vi "Elevator Controller.vi"(8 "error in":errorcluster) -> ()   [LabVIEW 2017]
doc: "This VI executes continuously carrying out the current operation and responding to updates or new operations. It will often contain the timing or control code that is difficult to place directly in TeleOp. This VI generally opens all sensors and motors and isolates the rest of the robot code from knowing how the operations are carried out."
uses:
  <vilib>/Rock Robotics/WPI/Framework/Completion Status.ctl
  Elevator Setpoints.ctl
  Elevator Operations.ctl
  <vilib>/Rock Robotics/WPI/ThirdParty/Phoenix-LabVIEW/Motor Controller/Controls/CTRE_Phoenix_MotorControl_FeedbackDevice.ctl
  <vilib>/Rock Robotics/WPI/ThirdParty/Phoenix-LabVIEW/Motor Controller/Controls/CTRE_Phoenix_MotorControl_LimitSwitchSource_Local.ctl
  <vilib>/Rock Robotics/WPI/ThirdParty/Phoenix-LabVIEW/Motor Controller/Controls/CTRE_Phoenix_MotorControl_LimitSwitchNormal.ctl
  <vilib>/Rock Robotics/WPI/ThirdParty/Phoenix-LabVIEW/Motor Controller/Controls/CTRE_Phoenix_MotorControl_ControlMode.ctl
  <vilib>/Rock Robotics/WPI/ThirdParty/Phoenix-LabVIEW/Motor Controller/Get/CTRE_Phoenix_MotorController_GetOutputCurrent_Enhanced.vi
  <vilib>/Rock Robotics/WPI/ThirdParty/Phoenix-LabVIEW/Motor Controller/Get/CTRE_Phoenix_MotorController_GetVoltage.vi
  Support Code/Global Constants.vi
  <vilib>/Rock Robotics/WPI/ThirdParty/Phoenix-LabVIEW/Motor Controller/Get/CTRE_Phoenix_MotorController_GetSelectedSensorData.vi
  <vilib>/Rock Robotics/Network Tables/NT Write Boolean.vi
panel:
  out "Current":dbl=0.5
  out "Output":dbl=0.06256109481915934
  out "Current":dbl(graph)=0.5
  out "Output":dbl(graph)=0.06256109481915934
  in  "F":dbl=0.0095 format="%#_13g"
  in  "P":dbl=0.7 format="%#_13g"
  in  "Max Acceleration":i32=6000
  in  "Cruise Velocity":i32=6000
  in  "Interactive Values":T1={"Operation"=enum."Zero Elevator Encoders", "Setpoint"=2.0, "Duration"=0.0}
  out "Current\nCmd":string="Started at  09:56:44.845\n: Reserve,  S 0.0, D 0.000000"
  in  "Buttons":cluster{"Execute Cmd":bool, "Abort Cmd":bool}
  out "Command Timing":cluster{"Start Time (ms)":u32, "Iterations":i32}={"Start Time (ms)"=1100696, "Iterations"=0}
  out "Status":T3
  # "Interactive Command: You may fill in the settings for a command\nand schedule it with the Execute button. You can observe and abort\nany command while fine tuning the code for the controller."
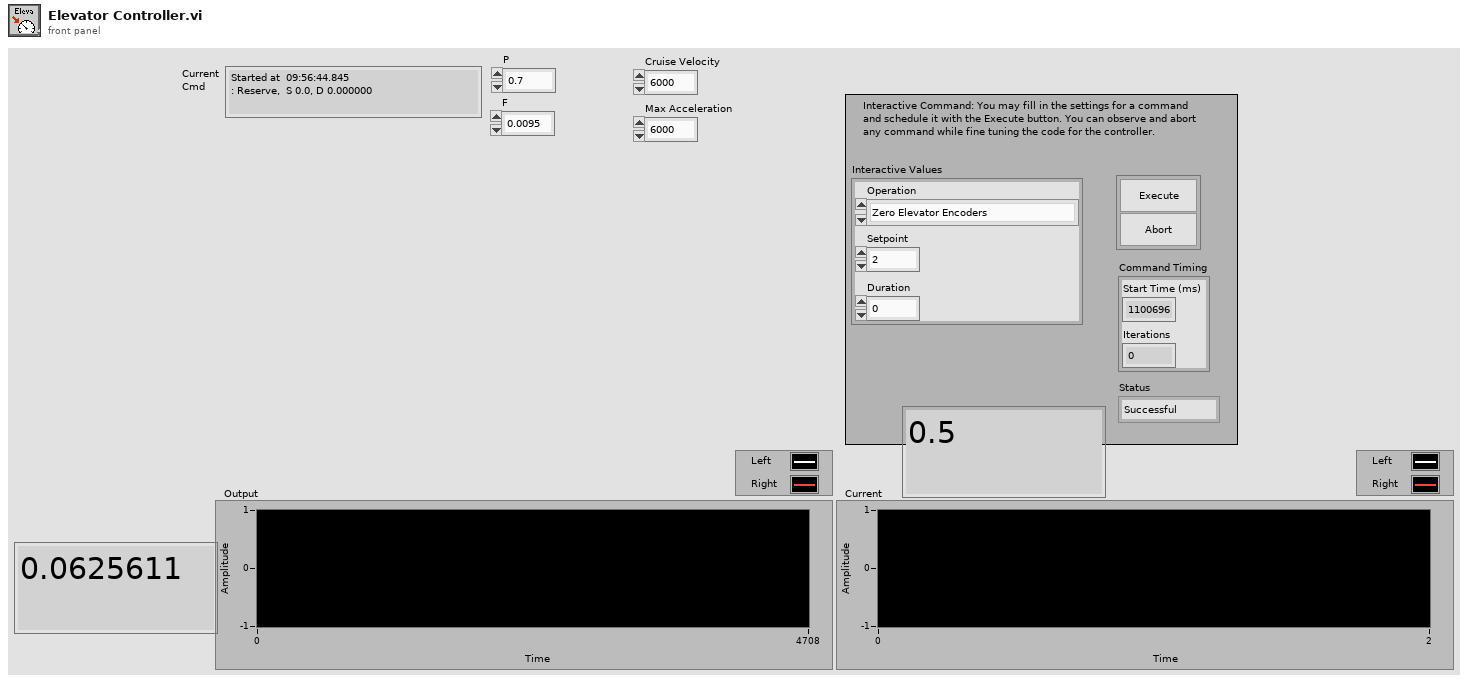
[diagram p1: front panel]
types:
  T1 = typedef "Elevator Setpoints.ctl" = cluster{"Operation":T2, "Setpoint":dbl, "Duration":dbl}
  T2 = typedef "Elevator Operations.ctl" = enum16{"Reserve", "Read Current", "Immediate", "Go to Height", "Fudge Up", "Fudge Down", "Zero Elevator Encoders", "Go to A", "Hold A", "Hold A for Duration"}
  T3 = typedef "Completion Status.ctl" = enum16{"Successful", "Aborted", "Incomplete"}
  T4 = typedef "CTRE_Phoenix_MotorControl_LimitSwitchNormal.ctl" = enum16{"Normally Open", "Normally Closed", "Disabled"}
  T5 = typedef "CTRE_Phoenix_MotorControl_LimitSwitchSource_Local.ctl" = enum16{"Feedback Connector", "Remote Talon SRX", "Remote CANifier", "Deactivated"}
  T6 = typedef "CTRE_Phoenix_MotorControl_FeedbackDevice.ctl" = i8
  T7 = typedef "WPI_MotorControlDeviceRef.ctl" = cluster{"DeviceStatus":errorcluster, "Type":T8, "PWM":cluster{"PWM Channel":T9, "DeadBand":T10}, "CAN":cluster{"Device Number":u8, "SetOutput VI Ref":variant, "GetOutput VI Ref":variant, "Enable VI Ref":variant, "Disable VI Ref":variant, "Data":variant}, "Invert":bool, "DIO PWM":cluster{"PWM \"Enable\" Channel":T9, "DIOChannel":T11, "PWM Rate":dbl}}
  T8 = typedef "WPI_MotorControlType.ctl" = enum16{"PWM", "CAN", "DIO PWM"}
  T9 = typedef "FPGA_DIOPWMChannel.ctl" = enum8{"PWM 0", "PWM 1", "PWM 2", "PWM 3", "PWM 4", "PWM 5", "PWM 6", "PWM 7", "PWM 8", "PWM 9", "PWM MXP 0", "PWM MXP 1", "PWM MXP 2", "PWM MXP 3", "PWM MXP 4", "PWM MXP 5", "PWM MXP 6", "PWM MXP 7", "PWM MXP 8", "PWM MXP 9", "Invalid"}
  T10 = typedef "WPI_PWMDeadband.ctl" = cluster{"Name":string, "maxPositivePwm":i32, "minPositivePwm":i32, "centerPwm":i32, "maxNegativePwm":i32, "minNegativePwm":i32, "angularRange":u16}
  T11 = typedef "FPGA_DIOChannel.ctl" = enum8{"DIO 0", "DIO 1", "DIO 2", "DIO 3", "DIO 4", "DIO 5", "DIO 6", "DIO 7", "DIO 8", "DIO 9", "DIO MXP 0", "DIO MXP 1", "DIO MXP 2", "DIO MXP 3", "DIO MXP 4", "DIO MXP 5", "DIO MXP 6", "DIO MXP 7", "DIO MXP 8", "DIO MXP 9", "DIO MXP 10", "DIO MXP 11", "DIO MXP 12", "DIO MXP 13", "DIO MXP 14", "DIO MXP 15", "SPI Port CS1", "SPI Port CS2", "SPI Port CS3", "SPI Port MISO", "SPI Port MOSI", "Invalid"}
  T12 = typedef "Command Status Info.ctl" = cluster{"Name":string, "Status":T3, "notifier out":T13}
  T13 = typedef "Completion Notifier.ctl" = refnum<notifier>
  T14 = cluster{"Current Command":T1, "Command Timing":cluster{"Start Time (ms)":u32, "Iterations":i32}, "Command Arguments":cluster{"Command Info":T12, "Description":string, "Default Command":T1, "queue out":refnum<queue>, "Subsystem Name":string}}
  T15 = typedef "CTRE_Phoenix_MotorControl_ControlMode.ctl" = u16
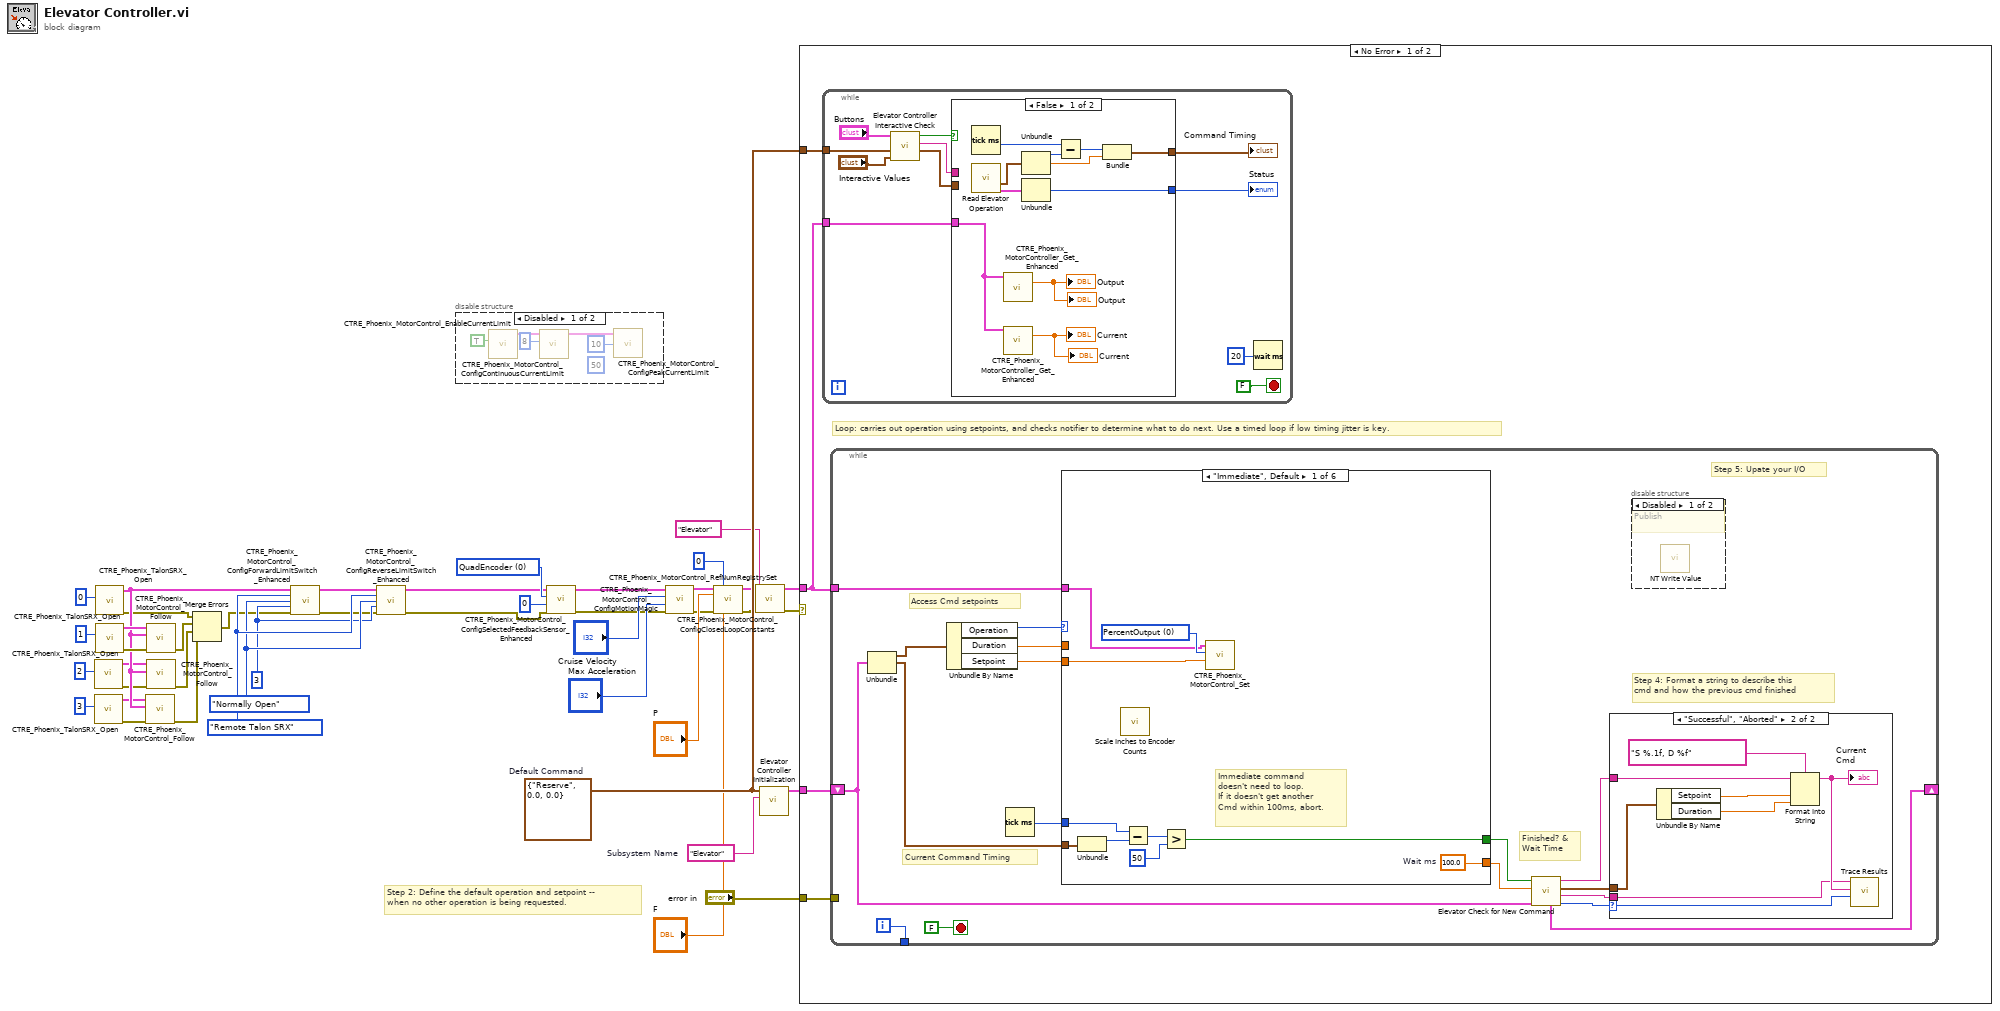
[diagram p0: block diagram]
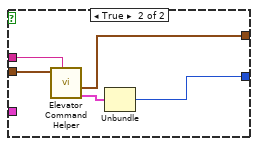
[diagram p2: hidden frame]
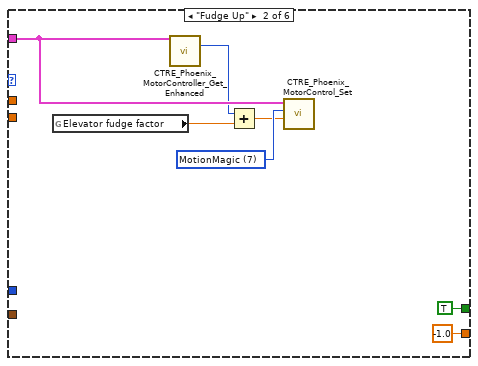
[diagram p5: hidden frame]
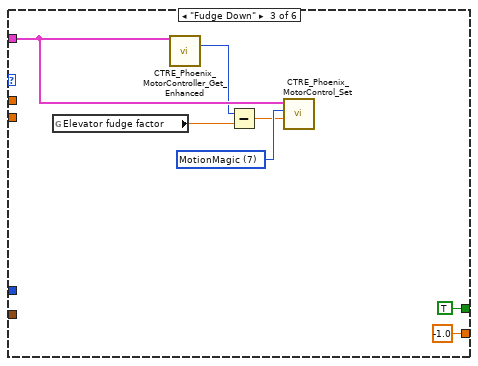
[diagram p6: hidden frame]
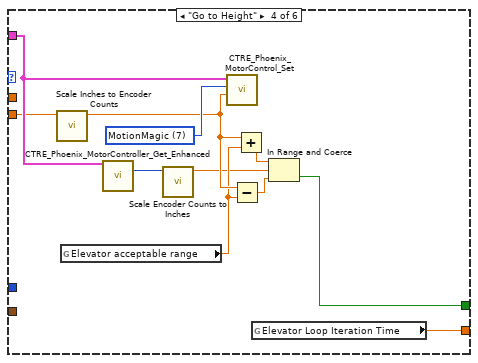
[diagram p7: hidden frame]
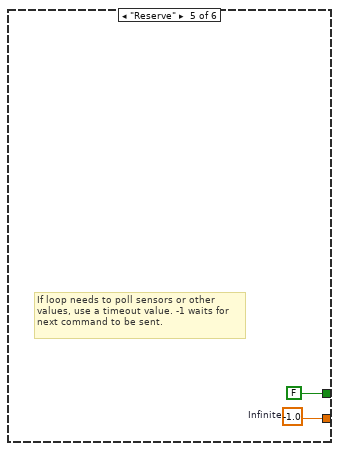
[diagram p8: hidden frame]
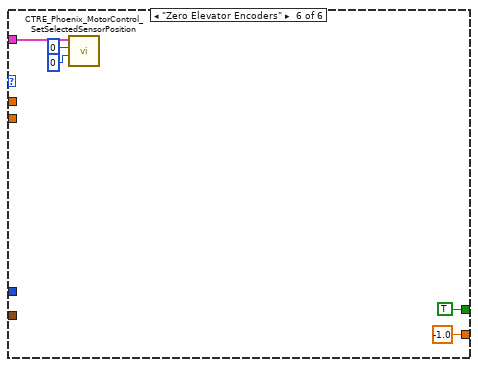
[diagram p9: hidden frame]
diagram:
  w21 = 3 ("deviceID")
  w22 = CTRE_Phoenix_MotorControl_LimitSwitchNormal."Normally Open" ("NormallyOpenOrClosed")
  w23 = CTRE_Phoenix_MotorControl_LimitSwitchSource_Local."Remote Talon SRX" ("Limit Switch Source")
  w27 = T6 0 items=["None"=-1, "QuadEncoder"=0, "Analog"=2, "Tachometer"=4, "Pulse Width Encoded Position"=8, "Sensor Sum (S0 + S1)"=9, "Sensor Difference (D0 - D1)"=10, "Remote Source 0"=11, "Remote Source 1"=12, "Software Emulated"=15] ("Feedback Device")
  w40 = T1 {"Operation"=enum."Reserve", "Setpoint"=0.0, "Duration"=0.0}  # Default Command
  w41 = "Elevator"  # Subsystem Name
  # "Step 2: Define the default operation and setpoint --\nwhen no other operation is being requested."
  n1 = call <vilib>:"CTRE_Phoenix_TalonSRX_Open.vi"("Device Number"=u8 2) -> ("error out"=w4:errorcluster, "CAN Talon SRX Ref"=w3:T7)  [unwired: 9 in]
  n2 = call <vilib>:"CTRE_Phoenix_TalonSRX_Open.vi"("Device Number"=u8 3) -> ("error out"=w2:errorcluster, "CAN Talon SRX Ref"=w1:T7)  [unwired: 9 in]
  n3 = call <vilib>:"CTRE_Phoenix_TalonSRX_Open.vi"("Device Number"=u8 0) -> ("error out"=w20:errorcluster, "CAN Talon SRX Ref"=w26:T7)  [unwired: 9 in]
  n4 = call <vilib>:"CTRE_Phoenix_TalonSRX_Open.vi"("Device Number"=u8 1) -> ("error out"=w30:errorcluster, "CAN Talon SRX Ref"=w29:T7)  [unwired: 9 in]
  n5 = call <vilib>:"CTRE_Phoenix_MotorControl_Follow.vi"("error in (no error)"=w2, "Master Controller to Follow"=w26, "PhoenixMotorControlDevRef"=w1) -> ("error out"=w17:errorcluster)  [unwired: 7 in, 1 out]
  n6 = call <vilib>:"CTRE_Phoenix_MotorControl_Follow.vi"("error in (no error)"=w30, "Master Controller to Follow"=w26, "PhoenixMotorControlDevRef"=w29) -> ("error out"=w19:errorcluster)  [unwired: 7 in, 1 out]
  n7 = call <vilib>:"CTRE_Phoenix_MotorControl_Follow.vi"("error in (no error)"=w4, "Master Controller to Follow"=w26, "PhoenixMotorControlDevRef"=w3) -> ("error out"=w18:errorcluster)  [unwired: 7 in, 1 out]
  n8 = Merge Errors(w20, w19, w18, w17) -> (w16:errorcluster)
  n9 = call <vilib>:"CTRE_Phoenix_MotorControl_ConfigForwardLimitSwitch_Enhanced.vi"("PhoenixMotorControlDevRef"=w26, "Limit Switch Source"=w23, "NormallyOpenOrClosed"=w22, "deviceID"=w21, "error in (no error)"=w16) -> ("PhoenixMotorControlDevRef"=w25:T7, "error out"=w15:errorcluster)  [unwired: 9 in]
  n10 = call <vilib>:"CTRE_Phoenix_MotorControl_ConfigReverseLimitSwitch_Enhanced.vi"("PhoenixMotorControlDevRef"=w25, "Limit Switch Source"=w23, "NormallyOpenOrClosed"=w22, "deviceID"=w21, "error in (no error)"=w15) -> ("PhoenixMotorControlDevRef"=w24:T7, "error out"=w14:errorcluster)  [unwired: 9 in]
  n11 = disable-structure shown="Disabled" {
    frame Disabled {
      (unwired) 50 ("Peak Current Maximum Duration (ms)")
      n12 = call <vilib>:"CTRE_Phoenix_MotorControl_EnableCurrentLimit.vi"("Enable Current Limit?"=TRUE) -> ("PhoenixMotorControlDevRef"=w47:T7)  [unwired: 9 in, 1 out]
      n13 = call <vilib>:"CTRE_Phoenix_MotorControl_ConfigContinuousCurrentLimit.vi"("Continuous Current Limit (Amps)"=8, "PhoenixMotorControlDevRef"=w47) -> ("PhoenixMotorControlDevRef"=w48:T7)  [unwired: 8 in, 1 out]
      n14 = call <vilib>:"CTRE_Phoenix_MotorControl_ConfigPeakCurrentLimit.vi"("Peak Current (Amps)"=10, "PhoenixMotorControlDevRef"=w48) -> ()  [unwired: 8 in, 2 out]
    }
    frame Enabled {
    }
  }
  n15 = call <vilib>:"CTRE_Phoenix_MotorControl_ConfigSelectedFeedbackSensor_Enhanced.vi"("error in (no error)"=w14, "pidLoopIdx"=0, "Feedback Device"=w27, "PhoenixMotorControlDevRef"=w24) -> ("error out"=w13:errorcluster, "PhoenixMotorControlDevRef"=w32:T7)  [unwired: 6 in]
  n16 = call <vilib>:"CTRE_Phoenix_MotorControl_ConfigMotionMagic.vi"("error in (no error)"=w13, "Acceleration"="Max Acceleration", "Cruise Velocity"="Cruise Velocity", "PhoenixMotorControlDevRef"=w32) -> ("error out"=w12:errorcluster, "PhoenixMotorControlDevRef"=w36:T7)  [unwired: 6 in]
  n17 = call <vilib>:"CTRE_Phoenix_MotorControl_ConfigClosedLoopConstants.vi"("PhoenixMotorControlDevRef"=w36, "slotIdx"=0, "P"="P", "error in (no error)"=w12, "F"="F") -> ("PhoenixMotorControlDevRef"=w10:T7, "error out"=w8:errorcluster)  [unwired: 9 in]
  n18 = call <vilib>:"CTRE_Phoenix_MotorControl_RefNumRegistrySet.vi"("error in (no error)"=w8, "refnum name"="Elevator", "PhoenixMotorControlDevRef"=w10) -> ("error out"=w9:errorcluster, "PhoenixMotorControlDevRef"=w11:T7)  [unwired: 7 in]
  n19 = call "Elevator Controller Initialization.vi"("Subsystem Name"=w41, "Default Command"=w40) -> ("Current Command"=w42:T14)  [unwired: 9 in]
  n20 = case shown="No Error" w9 {
    tunnel: "error in" -> [w52 _]
    tunnel: w42 -> [w51 _]
    tunnel: w40 -> [w50 _]
    tunnel: w11 -> [w49 _]
    frame No Error {
      # "Loop: carries out operation using setpoints, and checks notifier to determine what to do next. Use a timed loop if low timing jitter is key."
      n21 = while {
        tunnel: w50 -> [w60]
        tunnel: w49 -> [w53]
        stop <- FALSE stop-if-true
        n22 = call "Elevator Controller Interactive Check.vi"("Interactive Command in"="Interactive Values", "Default Command"=w60, "Buttons"="Buttons") -> ("Interactive Command out"=w57:T1, "Trace String"=w58:string, "Schedule"=w59:bool)  [unwired: 6 in]
        n23 = case shown="False" w59 {
          tunnel: [w74 w79] -> w56
          tunnel: w57 -> [_ w77]
          tunnel: [w70 w75] -> w55
          tunnel: w58 -> [_ w78]
          tunnel: w53 -> [w66 _]
          frame False {
            n24 = Tick Count (ms)() -> (millisecond timer value=w69:u32)
            n25 = call "Read Elevator Operation.vi"() -> ("Command Info"=w67:T12, "SubSystem Data"=w68:T1)  [unwired: 9 in, 1 out]
            n26 = call-poly <vilib>:"CTRE_Phoenix_MotorController_Get_Enhanced.vi"("PhoenixMotorControlDevRef"=w66) -> ("Percent Output"=→"Output" →"Output":dbl)  [unwired: 10 in, 4 out]
            n27 = call-poly <vilib>:"CTRE_Phoenix_MotorController_Get_Enhanced.vi"("PhoenixMotorControlDevRef"=w66) -> ("Output Current"=→"Current" →"Current":dbl)  [unwired: 12 in, 2 out]
            n28 = Unbundle(w68) -> ("Operation"=w73:T2, "Setpoint"=w71:dbl)  [unwired: 1 out]
            n29 = Unbundle(w67) -> ("Status"=w74:T3)  [unwired: 2 out]
            n30 = Subtract(x=w69, y=w73) -> (x-y=w72:u32)
            n31 = Bundle(w72, "Setpoint"=w71) -> (w70:cluster{u32, "Setpoint":dbl})  [unwired: 1 in]
          }
          frame True {
            n32 = call "Elevator Command Helper.vi"("Description"=w78, "SubSystem Data"=w77) -> ("Command Info Out"=w76:T12, "Command Timing"=w75:cluster{"Start Time (ms)":u32, "Iterations":i32})  [unwired: 7 in, 1 out]
            n33 = Unbundle(w76) -> ("Status"=w79:T3)  [unwired: 2 out]
          }
        }
        "Status" <- w56
        "Command Timing" <- w55
        n34 = Wait (ms)(milliseconds to wait=u32 20) -> ()  [unwired: 1 out]
      }
      n35 = while {
        shift-right: [w88] -> _
        shift-left: w51 -> [w81]
        tunnel: [w95] -> _
        tunnel: w52 -> [_]
        tunnel: w49 -> [w80]
        i -> [w95]
        stop <- FALSE stop-if-true
        # "Step 5: Upate your I/O"
        # "Step 4: Format a string to describe this\ncmd and how the previous cmd finished"
        # "Current Command Timing"
        # "Access Cmd setpoints"
        # "Finished? &\nWait Time"
        n36 = Unbundle(w81) -> ("Current Command"=w94:T1, "Command Timing"=w90:cluster{"Start Time (ms)":u32, "Iterations":i32})  [unwired: 1 out]
        n37 = Unbundle By Name(w94) -> ("Operation"=w93:T2, "Duration"=w92:dbl, "Setpoint"=w89:dbl)
        n38 = Tick Count (ms)() -> (millisecond timer value=w91:u32)
        n39 = case shown="\"Immediate\", Default" w93 {
          tunnel: [w114 -1.0 ("Infinite") -1.0 ("Infinite") w136 w141 -1.0 ("Infinite")] -> w86
          tunnel: [w108 TRUE ("ignore previous (F)") TRUE ("ignore previous (F)") w137 FALSE ("ignore previous (F)") TRUE ("ignore previous (F)")] -> w87
          tunnel: w90 -> [w110 _ _ _ _ _]
          tunnel: w92 -> [_ _ _ _ _ _]
          tunnel: w91 -> [w109 _ _ _ _ _]
          tunnel: w89 -> [w105 _ _ w135 _ _]
          tunnel: w80 -> [w106 w118 w125 w138 _ w145]
          frame "Immediate", Default {
            w107 = T15 0 items=["PercentOutput"=0, "Position"=1, "Velocity"=2, "Current"=3, "Follower"=5, "MotionProfile"=6, "MotionMagic"=7, "MotionMagicArc"=8, "MotionProfileArc"=10, "Disabled"=15] ("Control Mode")
            w114 = 100.0  # Wait ms
            # "Immediate command\ndoesn't need to loop.\nIf it doesn't get another\nCmd within 100ms, abort."
            n40 = Unbundle(w110) -> ("Start Time (ms)"=w113:u32)  [unwired: 1 out]
            n41 = call "Scale Inches to Encoder Counts.vi"() -> ()  [unwired: 11 in, 1 out]
            n42 = Subtract(x=w109, y=w113) -> (x-y=w112:u32)
            n43 = Greater?(x=w112, y=u8 50 ("Left Motor")) -> (0:w108:bool)
            n44 = call <vilib>:"CTRE_Phoenix_MotorControl_Set.vi"("Output"=w105, "Control Mode"=w107, "PhoenixMotorControlDevRef"=w106) -> ()  [unwired: 7 in, 2 out]
          }
          frame "Fudge Up" {
            w121 = T15 7 items=["PercentOutput"=0, "Position"=1, "Velocity"=2, "Current"=3, "Follower"=5, "MotionProfile"=6, "MotionMagic"=7, "MotionMagicArc"=8, "MotionProfileArc"=10, "Disabled"=15] ("Control Mode")
            n45 = global read "Global Constants.vi" "Elevator fudge factor"() -> (w115:dbl)
            n46 = call-poly <vilib>:"CTRE_Phoenix_MotorController_Get_Enhanced.vi"("PhoenixMotorControlDevRef"=w118) -> ("Position (Raw Sensor Units)"=w117:i32)  [unwired: 11 in, 3 out]
            n47 = Add(x=w117, y=w115) -> (x+y=w116:dbl)
            n48 = call <vilib>:"CTRE_Phoenix_MotorControl_Set.vi"("Output"=w116, "Control Mode"=w121, "PhoenixMotorControlDevRef"=w118) -> ()  [unwired: 7 in, 2 out]
          }
          frame "Fudge Down" {
            w128 = T15 7 items=["PercentOutput"=0, "Position"=1, "Velocity"=2, "Current"=3, "Follower"=5, "MotionProfile"=6, "MotionMagic"=7, "MotionMagicArc"=8, "MotionProfileArc"=10, "Disabled"=15] ("Control Mode")
            n49 = global read "Global Constants.vi" "Elevator fudge factor"() -> (w122:dbl)
            n50 = call-poly <vilib>:"CTRE_Phoenix_MotorController_Get_Enhanced.vi"("PhoenixMotorControlDevRef"=w125) -> ("Position (Raw Sensor Units)"=w124:i32)  [unwired: 11 in, 3 out]
            n51 = Subtract(x=w124, y=w122) -> (x-y=w123:dbl)
            n52 = call <vilib>:"CTRE_Phoenix_MotorControl_Set.vi"("Output"=w123, "Control Mode"=w128, "PhoenixMotorControlDevRef"=w125) -> ()  [unwired: 7 in, 2 out]
          }
          frame "Go to Height" {
            w139 = T15 7 items=["PercentOutput"=0, "Position"=1, "Velocity"=2, "Current"=3, "Follower"=5, "MotionProfile"=6, "MotionMagic"=7, "MotionMagicArc"=8, "MotionProfileArc"=10, "Disabled"=15] ("Control Mode")
            n53 = call "Scale Inches to Encoder Counts.vi"("Target Height (in)"=w135) -> ("Encoder Counts"=w133:dbl)  [unwired: 10 in]
            n54 = global read "Global Constants.vi" "Elevator acceptable range"() -> (w132:dbl)
            n55 = call-poly <vilib>:"CTRE_Phoenix_MotorController_Get_Enhanced.vi"("PhoenixMotorControlDevRef"=w138) -> ("Position (Raw Sensor Units)"=w130:i32)  [unwired: 11 in, 3 out]
            n56 = call "Scale Encoder Counts to Inches.vi"("Target Height (in)"=w130) -> ("Encoder Counts"=w129:dbl)  [unwired: 10 in]
            n57 = call <vilib>:"CTRE_Phoenix_MotorControl_Set.vi"("Output"=w133, "Control Mode"=w139, "PhoenixMotorControlDevRef"=w138) -> ()  [unwired: 7 in, 2 out]
            n58 = Subtract(x=w133, y=w132) -> (x-y=w134:dbl)
            n59 = Add(x=w133, y=w132) -> (x+y=w131:dbl)
            n60 = global read "Global Constants.vi" "Elevator Loop Iteration Time"() -> (w136:dbl)
            n61 = In Range and Coerce(upper limit=w131, x=w129, lower limit=w134) -> (In Range?=w137:bool)  [unwired: 1 out]
          }
          frame "Reserve" {
            w141 = -1.0  # Infinite
            # "If loop needs to poll sensors or other\nvalues, use a timeout value. -1 waits for\nnext command to be sent."
          }
          frame "Zero Elevator Encoders" {
            n62 = call <vilib>:"CTRE_Phoenix_MotorControl_SetSelectedSensorPosition.vi"("pidLoopIdx"=0, "New Sensor Position"=0, "PhoenixMotorControlDevRef"=w145) -> ()  [unwired: 7 in, 2 out]
          }
        }
        n63 = call "Elevator Check for New Command.vi"("Current Command"=w81, "Wait time (ms)"=w86, "Finished?"=w87) -> ("Completion"=w82:T3, "Subsystem Name"=w83:string, "Current Command"=w84:T1, "Initial Trace String"=w85:string, "NextCommand"=w88:T14)  [unwired: 4 in]
        n64 = case shown="\"Successful\", \"Aborted\"" w82 {
          selector: w82 -> [_ w104]
          tunnel: w85 -> [_ w100]
          tunnel: w84 -> [_ w101]
          tunnel: w83 -> [_ w97]
          frame "Incomplete", Default {
            # "Continuing current command"
          }
          frame "Successful", "Aborted" {
            # "Report and setup for next command"
            n65 = Unbundle By Name(w101) -> ("Setpoint"=w103:dbl, "Duration"=w98:dbl)
            n66 = Format Into String(format string="S %.1f, D %f", initial string=w100, w103, w98) -> (resulting string=w99:string)  [unwired: 1 in, 1 out]
            "Current\nCmd" <- w99
            n67 = call <vilib>:"Trace Results.vi"("Status of previous command"=w104, "Description"=w99, "Subsystem"=w97) -> ()  [unwired: 9 in]
          }
        }
        n68 = disable-structure shown="Disabled" {
          frame Disabled {
            # "Publish"
            n69 = call-poly <vilib>:"NT Write Value.vi"() -> ()  [unwired: 11 in, 1 out]
          }
          frame Enabled {
          }
        }
      }
    }
    frame Error {
    }
  }
